vi "TTA_Global_Working_Directory.vi"() -> ()   [LabVIEW 2016]
panel:
  out "Working Directory":path
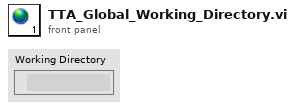
[diagram p1: front panel]
diagram:
